vi "Queue LogFile.vi"(4 "error in (no error)":errorcluster caption="Fehler (Eingang, kein Fehler)") -> (0 "error out":errorcluster caption="Fehler (Ausgang)", 3 "Queue (Ausgang)":refnum<queue>)   [LabVIEW 2020, in "LogKonfig.lvlib"]
uses:
  LogKonfig.lvlib
  FT-IR/TOOLweb Interface Library/TOOLweb Signalverlaeufe.ctl
  FT-IR/TOOLweb Interface Library/Typdefinitionen.lvlib
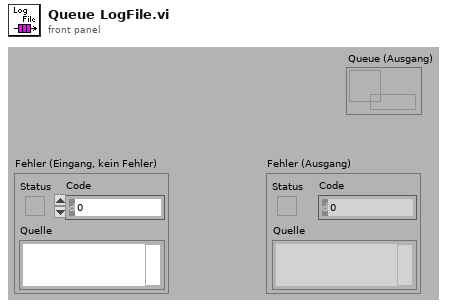
[diagram p1: front panel]
types:
  T1 = typedef "FT-IR.lvlib/TOOLweb Interface.lvlib/Typdefinitionen.lvlib/TOOLweb Signalverlaeufe.ctl" = waveform(dbl)[]
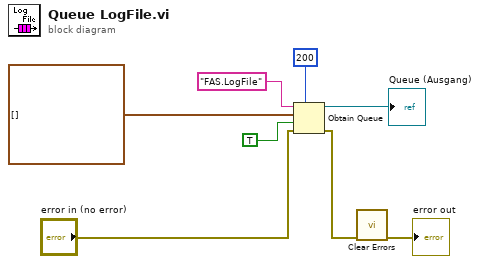
[diagram p0: block diagram]
diagram:
  n1 = Obtain Queue(max queue size (-1, unlimited)=200 ("Maximale Queue-Größe (-1, unbegrenzt)"), name (unnamed)="FAS.LogFile" ("Name (unbenannt)"), element data type=T1 [] ("Signalverläufe"), create if not found? (T)=TRUE ("Erzeugen, wenn nicht gefunden? (T)"), error in (no error)="error in (no error)") -> (queue out=→"Queue (Ausgang)":refnum<queue>, error out=w2:errorcluster)  [unwired: 1 out]
  n2 = call <vilib>:"Clear Errors.vi"("error in (no error)"=w2) -> ("error out"=→"error out":errorcluster)  [unwired: 5 in, 1 out]
